vi "delete object (SubVI).vi"(9 "contours in":T1(array[cluster]), 10 "output array in":string[][](array[string]), 11 "Object":i32) -> (1 "contours out":T1(array[cluster]), 2 "output array out":string[][](array[string]), 3 "Object":i32)   [LabVIEW 2020]
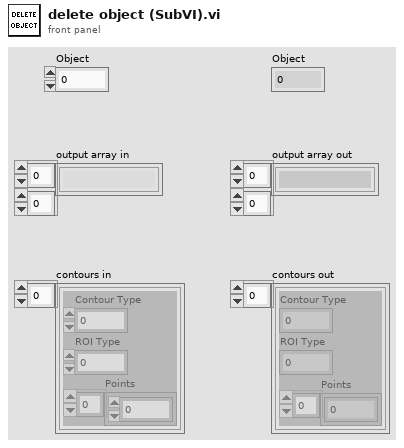
[diagram p1: front panel]
types:
  T1 = cluster{"Contour Type":u32, "ROI Type":u32, "Points":i32[]}[]
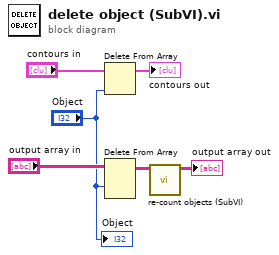
[diagram p0: block diagram]
diagram:
  n1 = Delete From Array(array="contours in", index="Object") -> (array with subset deleted=→"contours out":T1)  [unwired: 1 in, 1 out]
  n2 = Delete From Array(array="output array in", index (row)="Object") -> (array with subset deleted=w1:string[][])  [unwired: 2 in, 1 out]
  n3 = call "re-count objects (SubVI).vi"("output array in in"=w1) -> ("output array out"=→"output array out":string[][])  [unwired: 10 in]
  "Object" <- "Object"
